vi "PH_Beckhoff_StepMot.get Force Sensor Tagname.vi"(1 "Force Sensor Tag":T2, 2 "Force Sensor Location":T1) -> (0 "Force Sensor Tagname":string)   [LabVIEW 2014, in "PH_Beckhoff_StepMot.lvlib"]
doc: "This VI concatenates a Tagname out of strict type def enum controls. It keeps also the information whether the Tag is existing (if not, N/A is given out as name)."
uses:
  PH_Beckhoff_StepMot.lvlib
  PH_Beckhoff_StepMot.Force Sensor Tags.ctl
  PH_Beckhoff_StepMot.Force Sensor Location.ctl
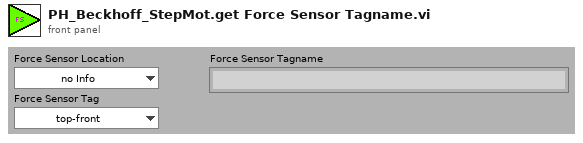
[diagram p1: front panel]
types:
  T1 = typedef "PH_Beckhoff_StepMot.lvlib/PH_Beckhoff_StepMot.Force Sensor Location.ctl" = enum16{"no Info", "MM1"}
  T2 = typedef "PH_Beckhoff_StepMot.lvlib/PH_Beckhoff_StepMot.Force Sensor Tags.ctl" = enum16{"top-front", "top-back", "bottom-front", "bottom-back"}
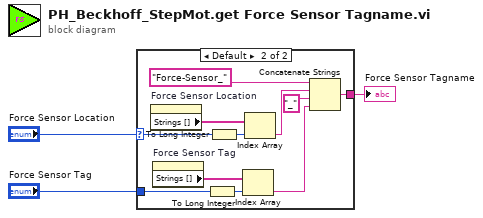
[diagram p0: block diagram]
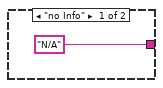
[diagram p2: hidden frame]
diagram:
  n1 = case shown="Default" "Force Sensor Location" {
    selector: "Force Sensor Location" -> [_ w12]
    tunnel: ["N/A" ("Subsystem_PU_Devices_Comm Type") w13] -> w2
    tunnel: "Force Sensor Tag" -> [_ w7]
    frame "no Info" {
    }
    frame Default {
      n2 = property on="Force Sensor Location" class="Enum (strict)"() -> ("Strings []"=w10:string[])  [unwired: 2 in, 2 out]
      n3 = property on="Force Sensor Tag" class="Enum (strict)"() -> ("Strings []"=w6:string[])  [unwired: 2 in, 2 out]
      n4 = To Long Integer(number=w7) -> (32bit integer=w8:i32)
      n5 = To Long Integer(number=w12) -> (32bit integer=w15:i32)
      n6 = Index Array(array=w6, index=w8) -> (element=w5:string)
      n7 = Index Array(array=w10, index=w15) -> (element=w14:string)
      n8 = Concatenate Strings("Force-Sensor_" ("string"), w14, "_" ("string"), w5) -> (w13:string)
    }
  }
  "Force Sensor Tagname" <- w2
